vi "CircularBuffer.SetCurrentElementIndex.vi"(8 "error in (no error)":errorcluster, 10 "Index":i32=1, 11 "CircularBuffer":refnum<class "CircularBuffer.lvclass">) -> (0 "error out":errorcluster, 3 "CircularBuffer out":refnum<class "CircularBuffer.lvclass">)   [LabVIEW 2016, in "CircularBuffer.lvclass"]
doc: "---------------------------------------------------------------\nJKI State Machine Objects™\nhttp://jki.net/state-machine-objects/\nCopyright (C) 2005-2015, JKI <info@jki.net>\nALL RIGHTS RESERVEDJKI State Machine Objects (SMO) 1.0.0.5\nJKI - JKI\nCopyright (c) 2016, JKI"
uses:
  CircularBuffer.lvclass
  CircularBuffer.lvclass/CircularBuffer.ctl
panel:
  # "For instructions on how to use the JKI State Machine Objects, examples and video tutorials, visit:\nhttp://jki.net/state-machine-objects/\n\nJKI State Machine Objects™\nhttp://jki.net/state-machine-objects/\nCopyright (C) 2005-2015, JKI <info@jki.net>\nALL RIGHTS RESERVED"
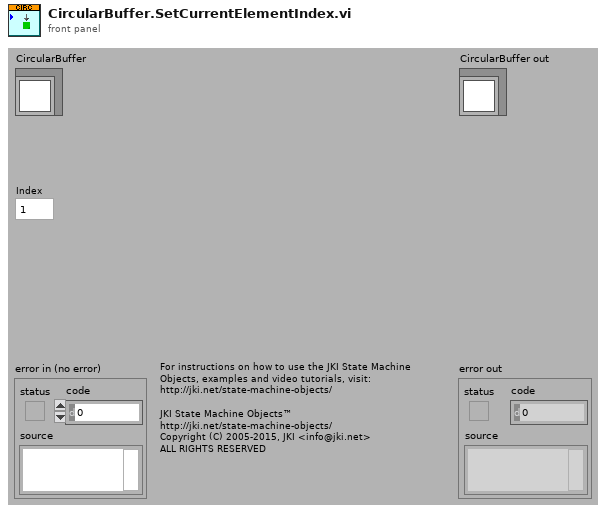
[diagram p1: front panel]
types:
  T1 = typedef "CircularBuffer.lvclass/PrivateData--Ref.ctl" = refnum<data-value>
  T2 = typedef "CircularBuffer.lvclass/PrivateData--Cluster.ctl" = cluster{"Public Events":T3, "Protected Events":T4, "Private Events":T5, "BufferSize":i32, "CurrentElement":i32, "Elements":refnum<data-value>[], "type":refnum<class "type.lvclass">}
  T3 = typedef "CircularBuffer.lvclass/PublicEvents--Cluster.ctl" = cluster{"Buffer Resize Event":refnum<user-event>}
  T4 = typedef "CircularBuffer.lvclass/ProtectedEvents--Cluster.ctl" = cluster{"placeholder":refnum<user-event>}
  T5 = typedef "CircularBuffer.lvclass/PrivateEvents--Cluster.ctl" = cluster{"New Value":refnum<user-event>, "GetElement":refnum<user-event>, "Initialize":refnum<user-event>}
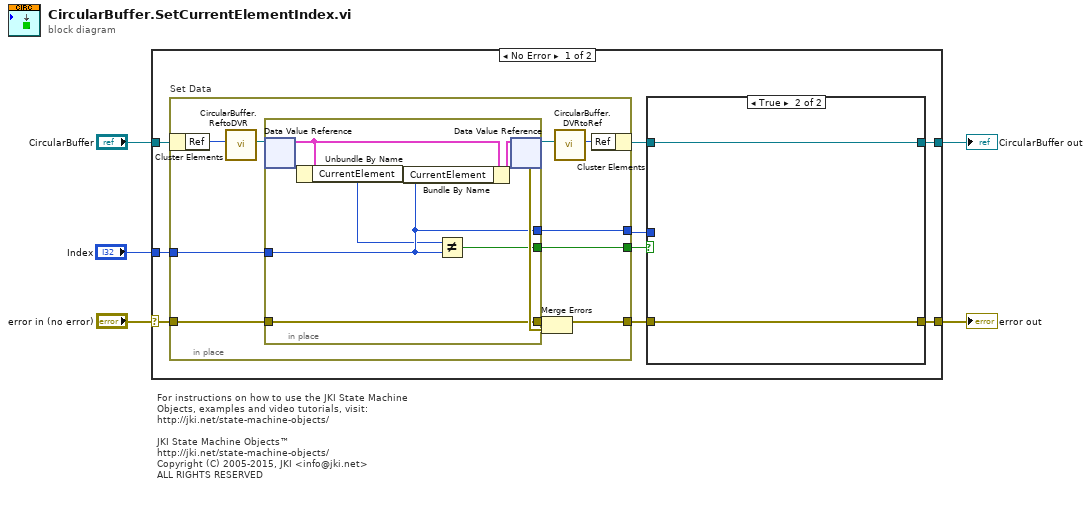
[diagram p0: block diagram]
diagram:
  # "For instructions on how to use the JKI State Machine Objects, examples and video tutorials, visit:\nhttp://jki.net/state-machine-objects/\n\nJKI State Machine Objects™\nhttp://jki.net/state-machine-objects/\nCopyright (C) 2005-2015, JKI <info@jki.net>\nALL RIGHTS RESERVED"
  n1 = case shown="No Error" "error in (no error)" {
    selector: "error in (no error)" -> [w12 w36]
    tunnel: "CircularBuffer" -> [w13 w37]
    tunnel: [w10 w36] -> w4
    tunnel: [w8 w37] -> w3
    tunnel: "Index" -> [w14 _]
    frame No Error {
      n2 = in-place "Set Data" {
        in-place-border: w12 -> [w29]
        in-place-border: [w26] -> w7
        in-place-border: w14 -> [w25]
        in-place-border: [w24] -> w11
        in-place-border: [w19] -> w6
        n3 = in-place-cluster #1(w13) -> ("Ref"=w23:u32)
        n4 = call "CircularBuffer.ReftoDVR.vi"("Ref"=w23) -> ("Ref"=w22:T1)  [unwired: 10 in]
        n5 = in-place {
          in-place-border: w29 -> [w35]
          in-place-border: [w35] -> w27
          in-place-border: w25 -> [w32]
          in-place-border: [w32] -> w24
          in-place-border: [w30] -> w19
          n6 = in-place-dvr #2(w22) -> (w33:T2)  [unwired: 1 out]
          n7 = Unbundle By Name(w33) -> ("CurrentElement"=w31:i32)
          n8 = Bundle By Name(cluster=w33, "CurrentElement"=w32) -> (w34:T2)
          n9 = Not Equal?(x=w31, y=w32) -> (x != y?=w30:bool)
          n10 = in-place-dvr #2(w34) -> (w21:T1, w28:errorcluster)
        }
        n11 = Merge Errors(w27, w28) -> (w26:errorcluster)
        n12 = call "CircularBuffer.DVRtoRef.vi"("Ref"=w21) -> ("Ref"=w20:u32)  [unwired: 10 in]
        n13 = in-place-cluster #1("Ref"=w20) -> (w9:refnum<class "CircularBuffer.lvclass">)
      }
      n14 = case shown="True" w6 {
        tunnel: w11 -> [_ _]
        tunnel: [w15 w17] -> w10
        tunnel: w9 -> [w16 w18]
        tunnel: [w16 w18] -> w8
        tunnel: w7 -> [w15 w17]
        frame False {
        }
        frame True {
        }
      }
    }
    frame Error {
    }
  }
  "error out" <- w4
  "CircularBuffer out" <- w3
